vi "projectfilenames.vi"(0 "Project Info":T1, 1 "Design Inputs":T2={"Q.Plant"=0.005, "C.CoagDoseMax"=0.01, "C.CoagStock"=0.015, "Ti.CoagStock"=0.0015, "EN.DrillSeries"=enum."English", "EN.TubeSeries"=enum."English", "N.SedTanks"=10.0, "N.SedBaysEst"=240.0, "W.SedPlate"=0.02, "L.SedPlateSheet"=0.0, "T.SedPlate"=388800000.0, "T.PlantWall"=0.03, "H.FlocOption"=0.01, "T.FlocBaffleRigidH"=0.03, "T.ConcreteMin"=0.3, "T.SedWeir"=0.3, "T.FlocBaffleRigidV"=108000.0} {"T.FlocBaffleRigidV" min=0.0 max=0.2 step=0.001 format="%#.1f"; "T.SedWeir" min=0.001 max=0.2 step=0.001 format="%#.1f"; "T.SedPlate" min=0.001 max=0.05 step=0.001 format="%#.1f"; "T.FlocBaffleRigidH" min=0.0 max=0.2 step=0.001 format="%#.1f"; "T.ConcreteMin" min=0.005 max=0.2 step=0.001 format="%#.1f"; "L.SedPlateSheet" min=0.3 max=8.0 step=0.01 format="%#.1f"; "N.SedBaysEst" min=1.0 max=20.0 step=1.0 format="%#.0f"; "N.SedTanks" min=1.0 max=20.0 step=1.0 format="%#.0f"; "Ti.CoagStock" min=43200.0 max=360000.0 step=3600.0 format="%#.1f"; "H.FlocOption" min=0.5 max=4.0 step=0.01 format="%#.2f"; "C.CoagStock" min=50.0 max=500.0 step=1.0 format="%#.0f"; "C.CoagDoseMax" min=0.03 max=0.2 step=0.005 format="%#.0f"; "Q.Plant" min=0.001 max=0.2 step=0.0001 format="%#.1f"; "T.PlantWall" min=0.05 max=0.5 step=0.001 format="%#.1f"; "W.SedPlate" min=0.5 max=3.0 step=0.001 format="%#.1f"}, 5 "Base File Path":path=path "C:/Documents and Settings/All Users/Documents/DesignData", 9 "User Information":T3 {"Country" items=["Afghanistan", "Aland Islands", "Albania", "Algeria", "American Samoa", "Andorra", "Angola", "Anguilla", "Antarctica", "Antigua And Barbuda", "Argentina", "Armenia", "Aruba", "Australia", "Austria", "Azerbaijan", "Bahamas", "Bahrain", "Bangladesh", "Barbados", "Belarus", "Belgium", "Belize", "Benin", "Bermuda", "Bhutan", "Bolivia", "Bosnia And Herzegovina", "Botswana", "Bouvet Island", "Brazil", "British Indian Ocean Territory", "Brunei Darussalam", "Bulgaria", "Burkina Faso", "Burundi", "Cambodia", "Cameroon", "Canada", "Cape Verde", "Cayman Islands", "Central African Republic", "Chad", "Chile", "China", "Christmas Island", "Cocos (Keeling) Islands", "Colombia", "Comoros", "Congo", "Congo, The Democratic Republic Of The", "Cook Islands", "Costa Rica", "Cote D'Ivoire", "Croatia", "Cuba", "Cyprus", "Czech Republic", "Denmark", "Djibouti", "Dominica", "Dominican Republic", "Ecuador", "Egypt", "El Salvador", "Equatorial Guinea", "Eritrea", "Estonia", "Ethiopia", "Falkland Islands (Malvinas)", "Faroe Islands", "Fiji", "Finland", "France", "French Guiana", "French Polynesia", "French Southern Territories", "Gabon", "Gambia", "Georgia", "Germany", "Ghana", "Gibraltar", "Greece", "Greenland", "Grenada", "Guadeloupe", "Guam", "Guatemala", "Guernsey", "Guinea", "Guinea-Bissau", "Guyana", "Haiti", "Heard Island And Mcdonald Islands", "Holy See (Vatican City State)", "Honduras", "Hong Kong", "Hungary", "Iceland", "India", "Indonesia", "Iran, Islamic Republic Of", "Iraq", "Ireland", "Isle Of Man", "Israel", "Italy", "Jamaica", "Japan", "Jersey", "Jordan", "Kazakhstan", "Kenya", "Kiribati", "Korea, Democratic People'S Republic Of", "Korea, Republic Of", "Kuwait", "Kyrgyzstan", "Lao People'S Democratic Republic", "Latvia", "Lebanon", "Lesotho", "Liberia", "Libyan Arab Jamahiriya", "Liechtenstein", "Lithuania", "Luxembourg", "Macao", "Macedonia, The Former Yugoslav Republic Of", "Madagascar", "Malawi", "Malaysia", "Maldives", "Mali", "Malta", "Marshall Islands", "Martinique", "Mauritania", "Mauritius", "Mayotte", "Mexico", "Micronesia, Federated States Of", "Moldova, Republic Of", "Monaco", "Mongolia", "Montserrat", "Morocco", "Mozambique", "Myanmar", "Namibia", "Nauru", "Nepal", "Netherlands", "Netherlands Antilles", "New Caledonia", "New Zealand", "Nicaragua", "Niger", "Nigeria", "Niue", "Norfolk Island", "Northern Mariana Islands", "Norway", "Oman", "Pakistan", "Palau", "Palestinian Territory, Occupied", "Panama", "Papua New Guinea", "Paraguay", "Peru", "Philippines", "Pitcairn", "Poland", "Portugal", "Puerto Rico", "Qatar", "Reunion", "Romania", "Russian Federation", "Rwanda", "Saint Helena", "Saint Kitts And Nevis", "Saint Lucia", "Saint Pierre And Miquelon", "Saint Vincent And The Grenadines", "Samoa", "San Marino", "Sao Tome And Principe", "Saudi Arabia", "Senegal", "Serbia And Montenegro", "Seychelles", "Sierra Leone", "Singapore", "Slovakia", "Slovenia", "Solomon Islands", "Somalia", "South Africa", "South Georgia And The South Sandwich Islands", "Spain", "Sri Lanka", "Sudan", "Suriname", "Svalbard And Jan Mayen", "Swaziland", "Sweden", "Switzerland", "Syrian Arab Republic", "Taiwan, Province Of China", "Tajikistan", "Tanzania, United Republic Of", "Thailand", "Timor-Leste", "Togo", "Tokelau", "Tonga", "Trinidad And Tobago", "Tunisia", "Turkey", "Turkmenistan", "Turks And Caicos Islands", "Tuvalu", "Uganda", "Ukraine", "United Arab Emirates", "United Kingdom", "United States", "United States Minor Outlying Islands", "Uruguay", "Uzbekistan", "Vanuatu", "Venezuela", "Viet Nam", "Virgin Islands, British", "Virgin Islands, U.S.", "Wallis And Futuna", "Western Sahara", "Yemen", "Zambia", "Zimbabwe", "(Not Specified)"]}, 11 "error in (no error)":errorcluster, 12 "Project command":T5=enum."New project", 13 "LstBox Refnum":refnum<vi>) -> (3 "Design Inputs out":T2={"Q.Plant"=0.0, "C.CoagDoseMax"=0.0, "C.CoagStock"=0.0, "Ti.CoagStock"=0.0, "EN.DrillSeries"=enum."English", "EN.TubeSeries"=enum."English", "N.SedTanks"=0.0, "N.SedBaysEst"=0.0, "W.SedPlate"=0.0, "L.SedPlateSheet"=0.0, "T.SedPlate"=0.0, "T.PlantWall"=0.03, "H.FlocOption"=0.01, "T.FlocBaffleRigidH"=0.03, "T.ConcreteMin"=0.3, "T.SedWeir"=0.3, "T.FlocBaffleRigidV"=108000.0} {"T.FlocBaffleRigidV" min=0.0 max=0.2 step=0.001 format="%#.1f"; "T.SedWeir" min=0.001 max=0.2 step=0.001 format="%#.1f"; "T.SedPlate" min=0.001 max=0.05 step=0.001 format="%#.1f"; "T.FlocBaffleRigidH" min=0.0 max=0.2 step=0.001 format="%#.1f"; "T.ConcreteMin" min=0.005 max=0.2 step=0.001 format="%#.1f"; "L.SedPlateSheet" min=0.3 max=8.0 step=0.01 format="%#.1f"; "N.SedBaysEst" min=1.0 max=20.0 step=1.0 format="%#.0f"; "N.SedTanks" min=1.0 max=20.0 step=1.0 format="%#.0f"; "Ti.CoagStock" min=43200.0 max=360000.0 step=3600.0 format="%#.1f"; "H.FlocOption" min=0.5 max=4.0 step=0.01 format="%#.2f"; "C.CoagStock" min=50.0 max=500.0 step=1.0 format="%#.0f"; "C.CoagDoseMax" min=0.03 max=0.2 step=0.005 format="%#.0f"; "Q.Plant" min=0.001 max=0.2 step=0.0001 format="%#.1f"; "T.PlantWall" min=0.05 max=0.5 step=0.001 format="%#.1f"; "W.SedPlate" min=0.5 max=3.0 step=0.001 format="%#.1f"}, 4 "File paths":T6, 8 "File List":string[](array[string]), 10 "Project Info out":T1, 14 "Project dates":timestamp[](array[timestamp]), 15 "error out":errorcluster)   [LabVIEW 2015, in "AguaClara Library.lvlib"]
uses:
  AguaClara Library.lvlib
  Project inputs.ctl
  File paths.ctl
  Project commands.ctl
  User Information.ctl
  Basic Inputs.ctl
  Country Ring.ctl
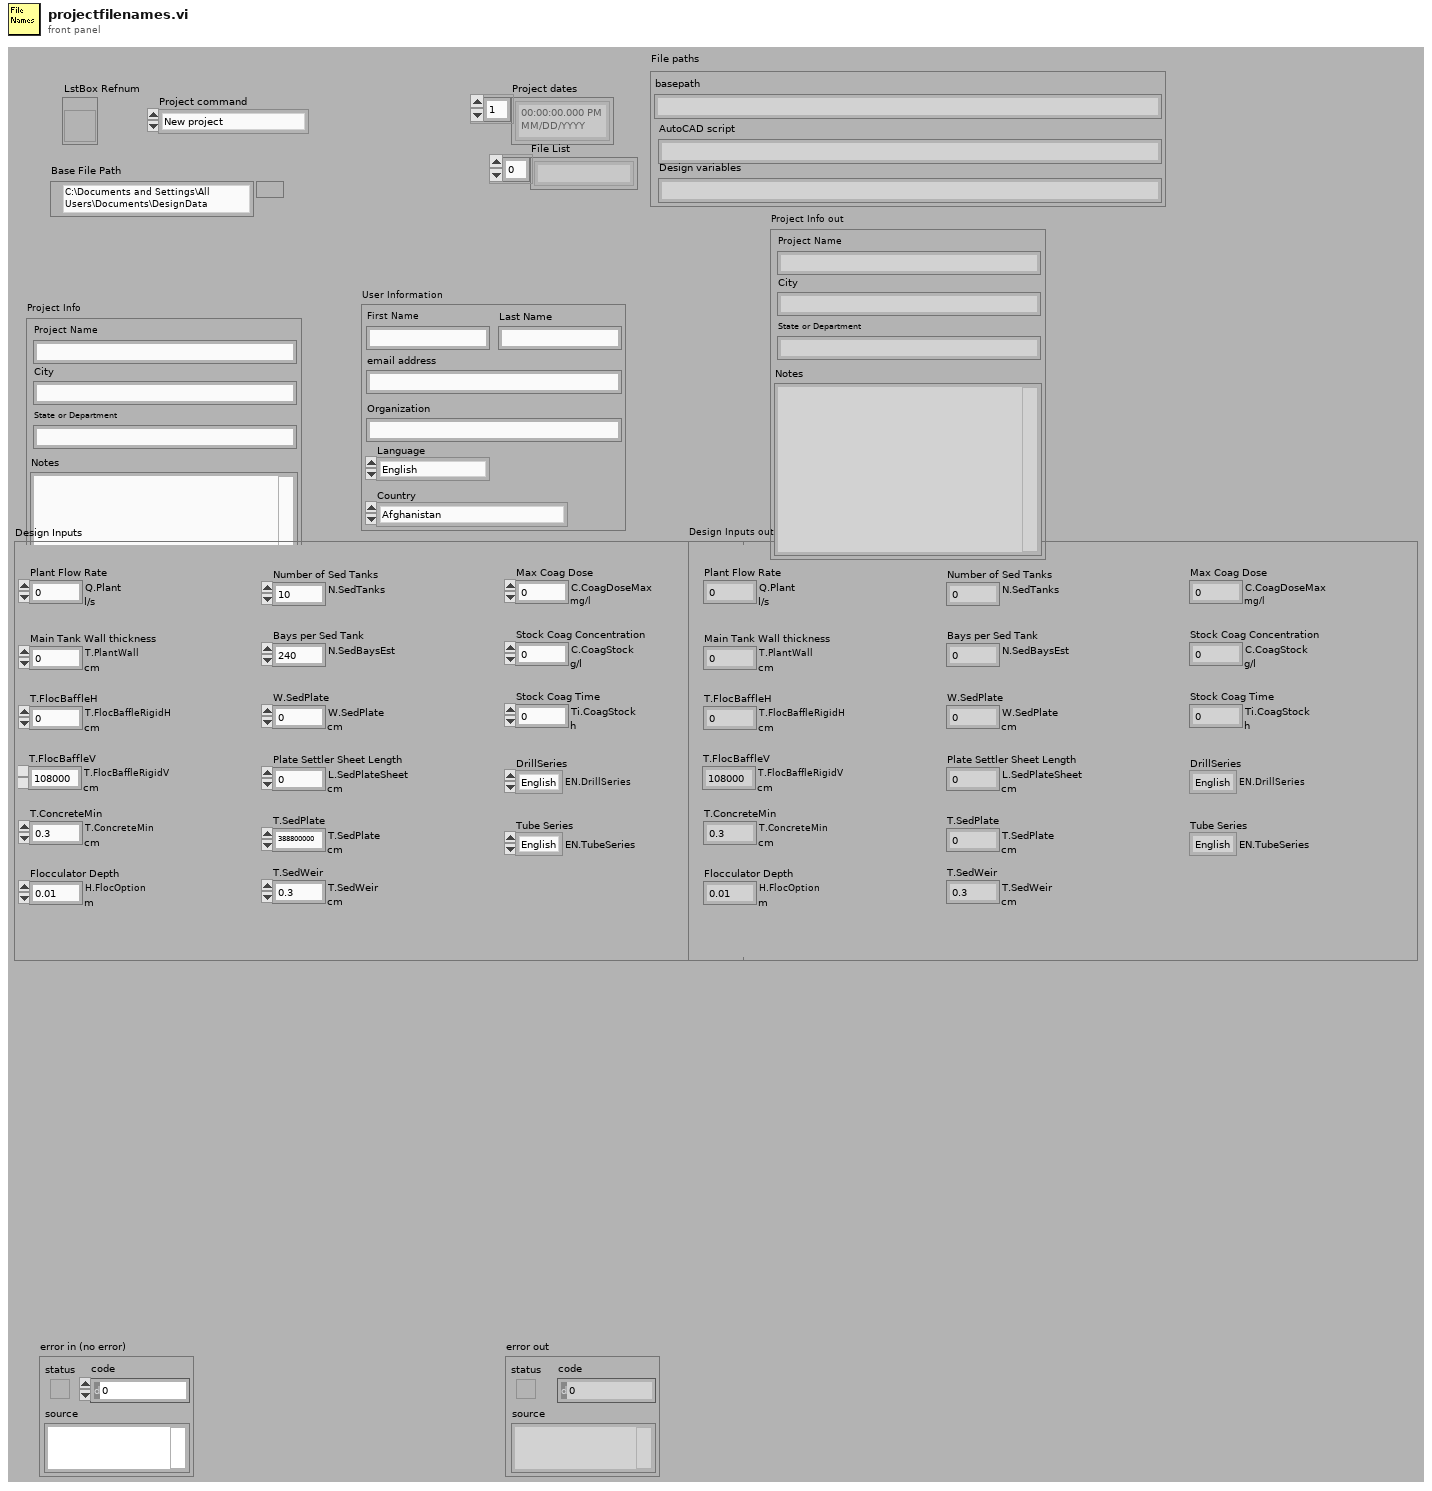
[diagram p1: front panel]
types:
  T1 = typedef "AguaClara Library.lvlib/Project inputs.ctl" = cluster{"Project Name":string, "City":string, "State":string, "Notes":string}
  T2 = typedef "AguaClara Library.lvlib/Basic Inputs.ctl" = cluster{"Q.Plant":dbl[unit], "C.CoagDoseMax":dbl[unit], "C.CoagStock":dbl[unit], "Ti.CoagStock":dbl[unit], "EN.DrillSeries":enum16{"English", "Metric"}, "EN.TubeSeries":enum16{"English", "Metric"}, "N.SedTanks":dbl, "N.SedBaysEst":dbl, "W.SedPlate":dbl[unit], "L.SedPlateSheet":dbl[unit], "T.SedPlate":dbl[unit], "T.PlantWall":dbl[unit], "H.FlocOption":dbl[unit], "T.FlocBaffleRigidH":dbl[unit], "T.ConcreteMin":dbl[unit], "T.SedWeir":dbl[unit], "T.FlocBaffleRigidV":dbl[unit]}
  T3 = typedef "AguaClara Library.lvlib/User Information.ctl" = cluster{"First Name":string, "Last Name":string, "Email Address":string, "Organization":string, "Language":enum16{"English", "Español", "French"}, "Country":T4}
  T4 = typedef "Country Ring.ctl" = u16
  T5 = typedef "AguaClara Library.lvlib/Project commands.ctl" = enum16{"Load base file", "Load User", "Read paths", "Open Project", "New project", "Edit project", "Delete project", "Mail project", "save design", "open design"}
  T6 = typedef "AguaClara Library.lvlib/File paths.ctl" = cluster{"basepath":string, "AutoCAD script":string, "Design variables":string}
  T7 = enum16{"open", "replace", "create", "open or create", "replace or create", "replace or create with confirmation"}
  T8 = typedef "Input Cluster.ctl" = cluster{"Project Info":T1, "Basic Inputs":T2}
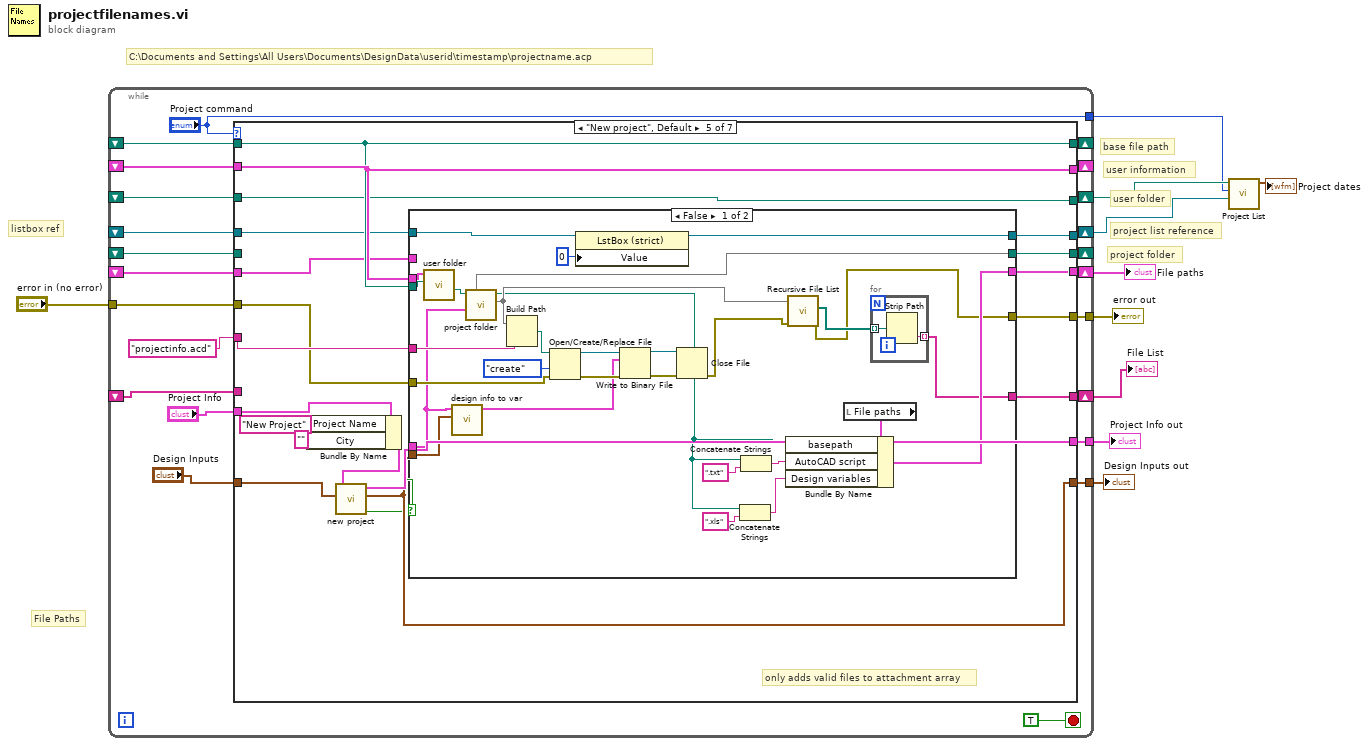
[diagram p0: block diagram]
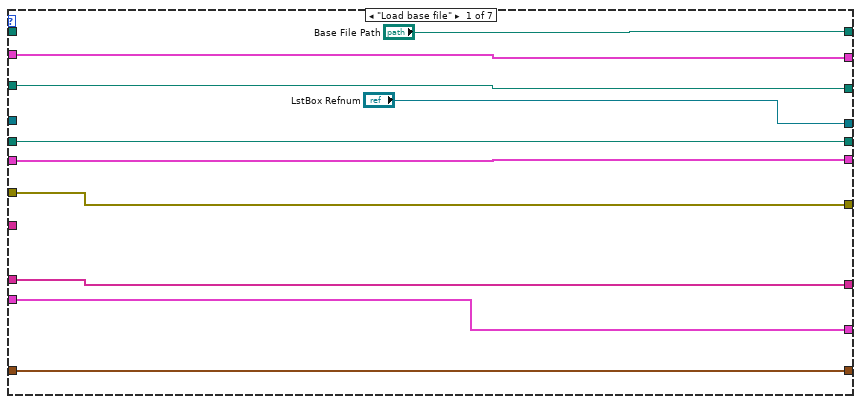
[diagram p2: hidden frame]
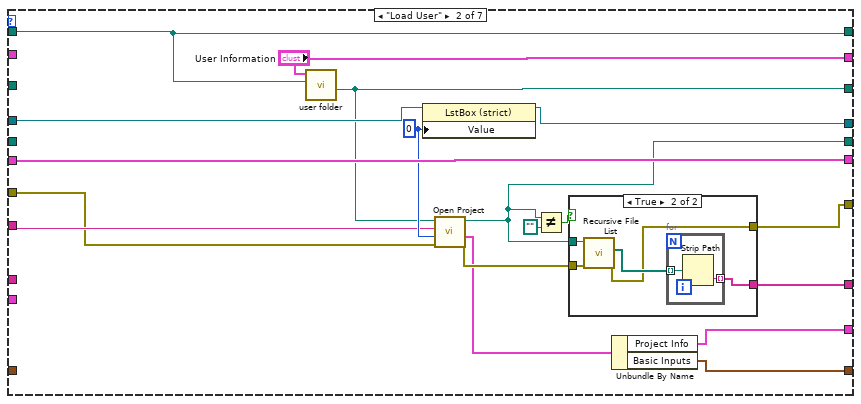
[diagram p3: hidden frame]
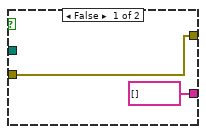
[diagram p4: hidden frame]
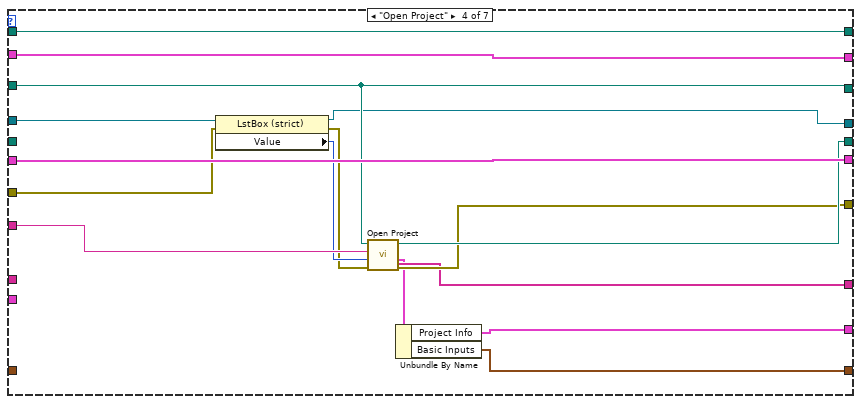
[diagram p6: hidden frame]
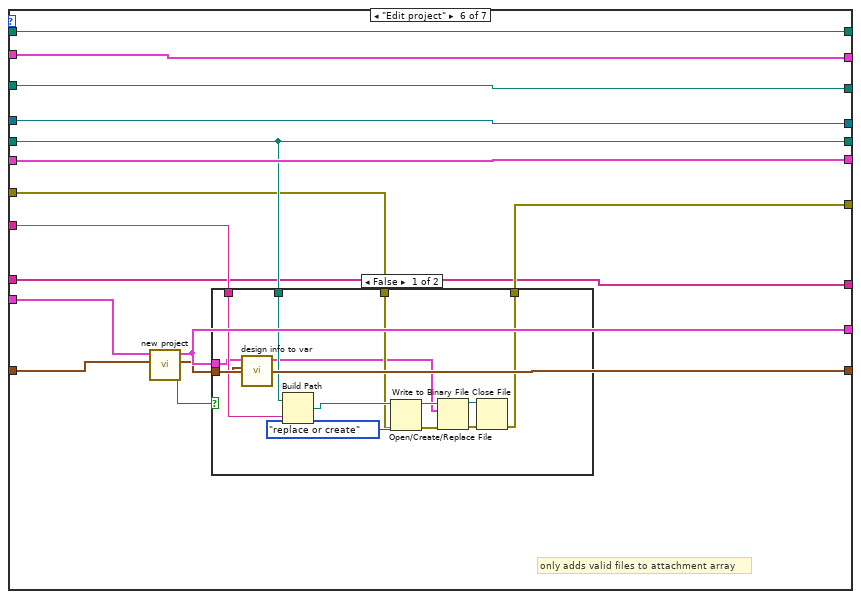
[diagram p8: hidden frame]
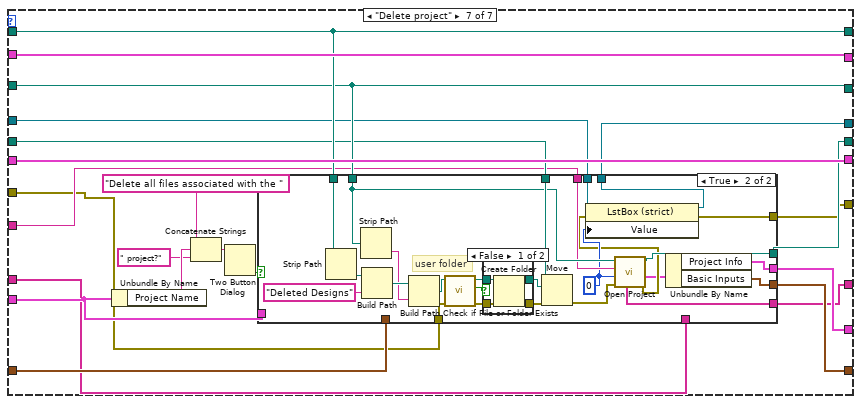
[diagram p10: hidden frame]
diagram:
  # "listbox ref"
  # "project list reference"
  # "project folder"
  # "user information"
  # "user folder"
  # "base file path"
  # "C:\\Documents and Settings\\All Users\\Documents\\DesignData\\userid\\timestamp\\projectname.acp"
  # "File Paths"
  n1 = while {
    shift-right: [w33] -> w10
    shift-left: _ -> [w32]
    shift-right: [w30] -> _
    shift-left: _ -> [w28]
    shift-right: [w29] -> _
    shift-left: _ -> [w27]
    shift-right: [w26] -> w7
    shift-left: _ -> [w25]
    tunnel: [w22] -> w9
    tunnel: [w21] -> w8
    shift-right: [w19] -> w4
    shift-left: _ -> [w18]
    shift-right: [w17] -> _
    shift-left: _ -> [w16]
    tunnel: ["Project command"] -> w5
    tunnel: "error in (no error)" -> [w14]
    tunnel: [w13] -> w2
    shift-right: [w12] -> w1
    shift-left: _ -> [w11]
    stop <- TRUE stop-if-true
    n2 = case shown="\"New project\", Default" "Project command" {
      tunnel: [w41 w61 w80 w94 w116 w162 w201] -> w33
      tunnel: w32 -> [w41 w61 w80 w94 w104 w162 w201]
      tunnel: ["Base File Path" w47 w79 w96 w114 w165 w200] -> w30
      tunnel: [w42 "User Information" w78 w95 w115 w166 w202] -> w29
      tunnel: w28 -> [_ w47 w79 w96 w114 w165 w200]
      tunnel: w27 -> [w42 _ w78 w95 w115 w166 w202]
      tunnel: [w40 w56 w76 w93 w113 w164 w194] -> w26
      tunnel: w25 -> [w40 _ w76 w93 w113 w164 w194]
      tunnel: "Design Inputs" -> [w38 _ w77 _ w110 w159 w187]
      tunnel: "Project Info" -> [w39 _ w75 _ w100 w161 w186]
      tunnel: [w39 w45 w75 w82 w111 w160 w188] -> w22
      tunnel: [w38 w44 w77 w81 w109 w158 w192] -> w21
      tunnel: "projectinfo.acd" ("name or relative path") -> [_ w55 _ w92 w112 w156 w190]
      tunnel: ["LstBox Refnum" w58 w74 w88 w106 w163 w189] -> w19
      tunnel: w18 -> [_ w59 w74 w89 w107 w163 w185]
      tunnel: [w37 w49 w73 w91 w108 w155 w191] -> w17
      tunnel: w16 -> [w37 _ w73 _ _ w155 w193]
      tunnel: w14 -> [w35 w54 w72 w86 w103 w154 w184]
      tunnel: [w35 w52 w72 w87 w102 w153 w183] -> w13
      tunnel: [w34 w51 w71 w84 w101 w152 w182] -> w12
      tunnel: w11 -> [w34 _ w71 _ _ w152 w181]
      frame "Load base file" {
      }
      frame "Load User" {
        w57 = 0 ("Value")
        n3 = call "user folder.vi"("Base File Path"=w47, "User Information"="User Information") -> ("User folder Path"=w56:path)  [unwired: 7 in, 2 out]
        n4 = property class="LstBox (strict)"(reference=w59, "Value"=w57) -> (reference out=w58:refnum<vi>)  [unwired: 1 in, 1 out]
        n5 = call "Open Project.vi"("error in (no error)"=w54, "project index"=w57, "name or relative path"=w55, "User folder Path"=w56) -> ("error out"=w53:errorcluster, "Input Cluster"=w46:T8, "Project Folder"=w49:path)  [unwired: 4 in, 1 out]
        n6 = Not Equal?(x=w49, y=path "") -> (x != y?=w48:bool)
        n7 = case shown="True" w48 {
          tunnel: w53 -> [w63 w67]
          tunnel: [w63 w66] -> w52
          tunnel: w49 -> [_ w65]
          tunnel: [string[] [] w64] -> w51
          frame False {
          }
          frame True {
            n8 = call <vilib>:"Recursive File List.vi"("error in (no error)"=w67, "Folder Path"=w65) -> ("error out"=w66:errorcluster, "All Files in Dir"=w68:path[])  [unwired: 5 in, 3 out]
            n9 = for {
              tunnel: w68 -> [w70] mode=indexing
              tunnel: [w69] -> w64 mode=indexing
              n10 = Strip Path(path=w70) -> (name=w69:string)  [unwired: 1 out]
            }
          }
        }
        n11 = Unbundle By Name(w46) -> ("Project Info"=w45:T1, "Basic Inputs"=w44:T2)
      }
      frame "Read paths" {
      }
      frame "Open Project" {
        n12 = property class="LstBox (strict)"(reference=w89, error in=w86) -> (reference out=w88:refnum<vi>, error out=w85:errorcluster, "Value"=w90:i32)
        n13 = call "Open Project.vi"("error in (no error)"=w85, "project index"=w90, "name or relative path"=w92, "User folder Path"=w93) -> ("error out"=w87:errorcluster, "Input Cluster"=w83:T8, "Project Folder"=w91:path, "File List"=w84:string[])  [unwired: 4 in]
        n14 = Unbundle By Name(w83) -> ("Project Info"=w82:T1, "Basic Inputs"=w81:T2)
      }
      frame "New project", Default {
        # "only adds valid files to attachment array"
        n15 = Bundle By Name(cluster=w100, "Project Name"="New Project", "City"="") -> (w99:T1)
        n16 = call "new project.vi"("Basic Inputs"=w110, "Project Info"=w99) -> ("canceled"=w105:bool, "Design Inputs out"=w109:T2, "Project Info out"=w111:T1)  [unwired: 7 in]
        n17 = case shown="False" w105 {
          tunnel: [w140 w149] -> w116
          tunnel: w115 -> [w139 _]
          tunnel: w114 -> [w138 w150]
          tunnel: w112 -> [w131 _]
          tunnel: w111 -> [w119 _]
          tunnel: w109 -> [w118 _]
          tunnel: [w122 w150] -> w108
          tunnel: w107 -> [w129 w151]
          tunnel: [w128 w151] -> w106
          tunnel: w104 -> [_ w149]
          tunnel: w103 -> [w126 w148]
          tunnel: [w123 w148] -> w102
          tunnel: [w121 _] -> w101
          frame False {
            n18 = call "user folder.vi"("Base File Path"=w138, "User Information"=w139) -> ("User folder Path"=w137:path)  [unwired: 7 in, 2 out]
            n19 = call "design info to var.vi"("Design Inputs"=w118, "Project Info"=w119) -> ("Array to save"=w117:cluster{"Label.Text":string, "Value":variant}[])  [unwired: 9 in]
            n20 = call "project folder.vi"("Request File Name"=w119, "Method"=w137) -> (2:w122, "Completed Design path"=w120:path)  [unwired: 7 in, 1 out]
            n21 = Build Path(base path=w122, name or relative path=w131) -> (appended path=w130:path)
            n22 = Open/Create/Replace File(file path (use dialog)=w130, error in=w126, operation (0:open)=T7."create") -> (refnum out=w134:refnum<file>, error out=w136:errorcluster)  [unwired: 3 in, 1 out]
            n23 = property class="LstBox (strict)"(reference=w129, "Value"=0) -> (reference out=w128:refnum<vi>)  [unwired: 1 in, 1 out]
            n24 = Write to Binary File(file (use dialog)=w134, data=w117, error in=w136) -> (refnum out=w132:refnum<file>, error out=w133:errorcluster)  [unwired: 3 in, 1 out]
            n25 = Close File(refnum=w132, error in=w133) -> (error out=w124:errorcluster)  [unwired: 1 out]
            n26 = Concatenate Strings(w120, ".xls" ("string")) -> (w141:string)
            n27 = Concatenate Strings(w120, ".txt" ("string")) -> (w144:string)
            n28 = call <vilib>:"Recursive File List.vi"("error in (no error)"=w124, "Folder Path"=w122) -> ("error out"=w123:errorcluster, "All Files in Dir"=w125:path[])  [unwired: 5 in, 3 out]
            n29 = local read "File paths"() -> (w142:T6)
            n30 = Bundle By Name(cluster=w142, "basepath"=w120, "AutoCAD script"=w144, "Design variables"=w141) -> (w140:T6)
            n31 = for {
              tunnel: w125 -> [w147] mode=indexing
              tunnel: [w146] -> w121 mode=indexing
              n32 = Strip Path(path=w147) -> (name=w146:string)  [unwired: 1 out]
            }
          }
          frame True {
          }
        }
      }
      frame "Edit project" {
        # "only adds valid files to attachment array"
        n33 = call "new project.vi"("Basic Inputs"=w159, "Project Info"=w161) -> ("canceled"=w157:bool, "Design Inputs out"=w158:T2, "Project Info out"=w160:T1)  [unwired: 7 in]
        n34 = case shown="False" w157 {
          tunnel: w160 -> [w169 _]
          tunnel: w158 -> [w168 _]
          tunnel: w155 -> [w174 _]
          tunnel: w156 -> [w173 _]
          tunnel: w154 -> [w171 w180]
          tunnel: [w170 w180] -> w153
          frame False {
            n35 = call "design info to var.vi"("Design Inputs"=w168, "Project Info"=w169) -> ("Array to save"=w167:cluster{"Label.Text":string, "Value":variant}[])  [unwired: 9 in]
            n36 = Build Path(base path=w174, name or relative path=w173) -> (appended path=w172:path)
            n37 = Open/Create/Replace File(file path (use dialog)=w172, error in=w171, operation (0:open)=T7."replace or create") -> (refnum out=w177:refnum<file>, error out=w179:errorcluster)  [unwired: 3 in, 1 out]
            n38 = Write to Binary File(file (use dialog)=w177, data=w167, error in=w179) -> (refnum out=w175:refnum<file>, error out=w176:errorcluster)  [unwired: 3 in, 1 out]
            n39 = Close File(refnum=w175, error in=w176) -> (error out=w170:errorcluster)  [unwired: 1 out]
          }
          frame True {
          }
        }
      }
      frame "Delete project" {
        n40 = Unbundle By Name(w186) -> ("Project Name"=w197:string)
        n41 = Concatenate Strings("Delete all files associated with the " ("message"), w197, " project?" ("string")) -> (w195:string)
        n42 = Two Button Dialog(message=w195) -> (T button?=w199:bool)  [unwired: 2 in]
        n43 = case shown="True" w199 {
          tunnel: w193 -> [w208 w233]
          tunnel: w200 -> [_ w227]
          tunnel: w194 -> [_ w223]
          tunnel: [w207 w209] -> w192
          tunnel: [w208 w224] -> w191
          tunnel: w190 -> [_ w219]
          tunnel: [w205 w217] -> w189
          tunnel: [w206 w210] -> w188
          tunnel: w187 -> [w207 _]
          tunnel: w186 -> [w206 _]
          tunnel: w185 -> [w205 w218]
          tunnel: w184 -> [w204 w215]
          tunnel: [w204 w213] -> w183
          tunnel: [w203 w212] -> w182
          tunnel: w181 -> [w203 _]
          frame False {
          }
          frame True {
            w216 = 0 ("project index")
            # "user folder"
            n44 = Strip Path(path=w227) -> (stripped path=w226:path)  [unwired: 1 out]
            n45 = Strip Path(path=w223) -> (name=w228:string)  [unwired: 1 out]
            n46 = Build Path(base path=w226, name or relative path="Deleted Designs") -> (appended path=w232:path)
            n47 = Build Path(base path=w232, name or relative path=w228) -> (appended path=w229:path)
            n48 = call <vilib>:"Check if File or Folder Exists.vi"("error in (no error)"=w215, "path"=w229) -> ("error out"=w220:errorcluster, "file or folder exists?"=w231:bool, "dup path"=w230:path)  [unwired: 7 in]
            n49 = case shown="False" w231 {
              tunnel: w230 -> [w238 w240]
              tunnel: [w237 w240] -> w225
              tunnel: [w236 w239] -> w221
              tunnel: w220 -> [w235 w239]
              frame False {
                n50 = Create Folder(path (use dialog)=w238, error in=w235) -> (created path=w237:path, error out=w236:errorcluster)  [unwired: 1 in, 1 out]
              }
              frame True {
              }
            }
            n51 = Move(source path=w233, error in=w221, 10:w225) -> (error out=w222:errorcluster)  [unwired: 2 in, 2 out]
            n52 = call "Open Project.vi"("error in (no error)"=w222, "project index"=w216, "name or relative path"=w219, "User folder Path"=w223) -> ("error out"=w214:errorcluster, "Input Cluster"=w211:T8, "Project Folder"=w224:path, "File List"=w212:string[])  [unwired: 4 in]
            n53 = property class="LstBox (strict)"(reference=w218, error in=w214, "Value"=w216) -> (reference out=w217:refnum<vi>, error out=w213:errorcluster)
            n54 = Unbundle By Name(w211) -> ("Project Info"=w210:T1, "Basic Inputs"=w209:T2)
          }
        }
      }
    }
  }
  "File paths" <- w10
  "Project Info out" <- w9
  "Design Inputs out" <- w8
  "error out" <- w2
  "File List" <- w1
  n55 = call "Project List.vi"("LstBox Refnum"=w4, "Project command"=w5, "User folder Path"=w7) -> ("Project dates"=→"Project dates":timestamp[])  [unwired: 3 in, 1 out]
